vi "set_rep_param.vi"(4 "error in (no error)":errorcluster, 5 "par_val":string, 6 "param_name":string, 7 "refnum":T1) -> (0 "error out":errorcluster, 3 "refnum out":T1)   [LabVIEW 2010]
uses:
  <vilib>/Utility/config.llb/Config Data RefNum.ctl
  <vilib>/Utility/config.llb/Write Key (I32).vi
  <vilib>/Utility/config.llb/Write Key (String).vi
  <vilib>/Utility/config.llb/Read Key (String).vi
  <vilib>/Utility/config.llb/NI_LVConfig.lvlib
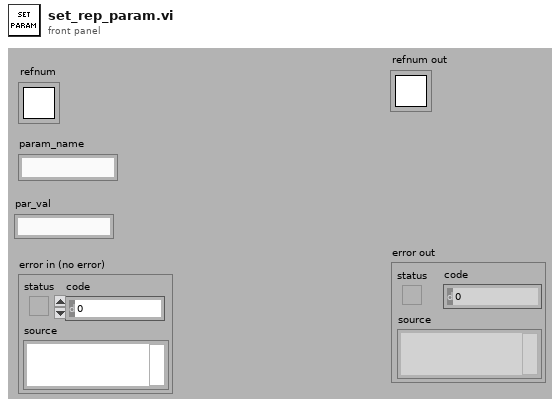
[diagram p1: front panel]
types:
  T1 = typedef "NI_LVConfig.lvlib/Config Data RefNum.ctl" = refnum<k1>
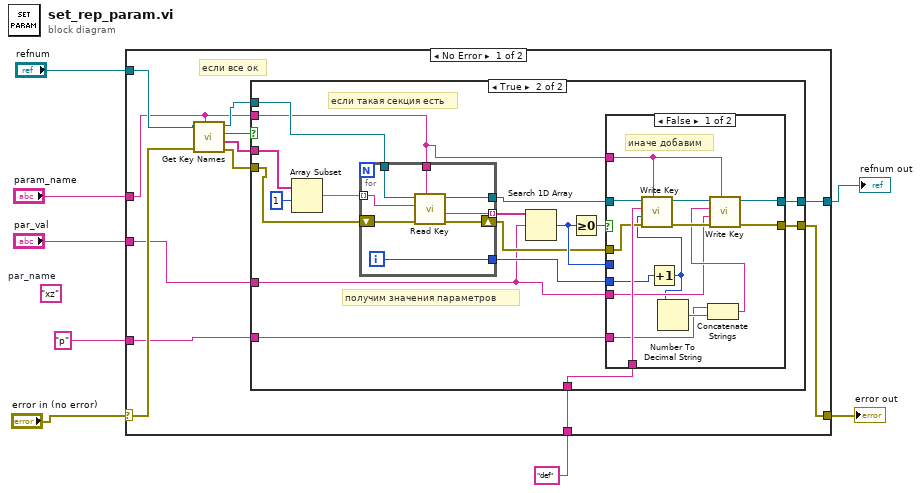
[diagram p0: block diagram]
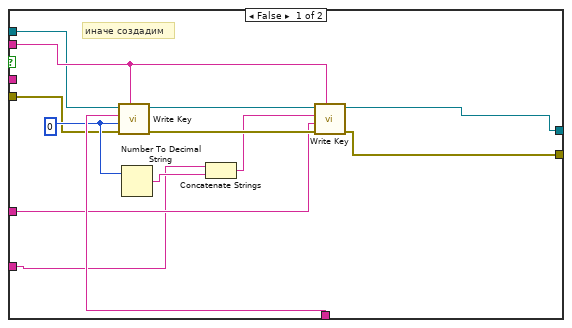
[diagram p2: hidden frame]
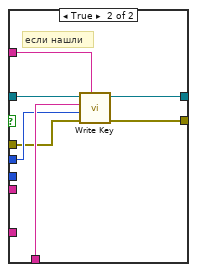
[diagram p3: hidden frame]
diagram:
  (unwired) "xz"  # par_name
  n1 = case shown="No Error" "error in (no error)" {
    selector: "error in (no error)" -> [w20 w81]
    tunnel: [w10 w81] -> w7
    tunnel: "refnum" -> [w19 w80]
    tunnel: "param_name" -> [w13 _]
    tunnel: "p" -> [w14 _]
    tunnel: "par_val" -> [w12 _]
    tunnel: "def" -> [w11 _]
    tunnel: [w9 w80] -> w1
    frame No Error {
      # "если все ок"
      n2 = call <vilib>:"Get Key Names.vi"("section"=w13, "error in (no error)"=w20, "refnum"=w19) -> ("error out"=w17:errorcluster, "key names"=w15:string[], "section exists?"=w18:bool, "refnum out"=w16:T1)  [unwired: 5 in]
      n3 = case shown="True" w18 {
        tunnel: w17 -> [w21 w48]
        tunnel: w16 -> [w30 w46]
        tunnel: w15 -> [_ w50]
        tunnel: w14 -> [w23 w37]
        tunnel: w13 -> [w31 w43]
        tunnel: w12 -> [w26 w36]
        tunnel: w11 -> [w27 w41]
        tunnel: [w28 w35] -> w10
        tunnel: [w29 w34] -> w9
        frame False {
          w25 = 0
          # "иначе создадим"
          n4 = call-poly <vilib>:"Write Key.vi"("section"=w31, "error in (no error)"=w21, "value"=w25, "key"=w27, "refnum"=w30) -> ("error out"=w33:errorcluster, "refnum out"=w32:T1)  [unwired: 4 in, 1 out]
          n5 = Number To Decimal String(number=w25) -> (decimal integer string=w24:string)  [unwired: 1 in]
          n6 = Concatenate Strings(w23, w24) -> (w22:string)
          n7 = call-poly <vilib>:"Write Key.vi"("section"=w31, "error in (no error)"=w33, "value"=w26, "key"=w22, "refnum"=w32) -> ("error out"=w28:errorcluster, "refnum out"=w29:T1)  [unwired: 4 in, 1 out]
        }
        frame True {
          # "получим значения параметров"
          # "если такая секция есть"
          n8 = Array Subset(array=w50, index=1) -> (w47:string[])  [unwired: 1 in]
          n9 = for {
            tunnel: w47 -> [w76] mode=indexing
            tunnel: w43 -> [w78]
            tunnel: w46 -> [w77]
            tunnel: [w74] -> w42
            tunnel: [w73] -> w45 mode=indexing
            shift-right: [w75] -> w39
            shift-left: w48 -> [w79]
            tunnel: [w72] -> w38
            i -> [w72]
            n10 = call-poly <vilib>:"Read Key.vi"("section"=w78, "error in (no error)"=w79, "key"=w76, "refnum"=w77) -> ("error out"=w75:errorcluster, "value"=w73:string, "refnum out"=w74:T1)  [unwired: 4 in, 1 out]
          }
          n11 = Search 1D Array(1D array=w45, element=w36) -> (index of element=w40:i32)  [unwired: 1 in]
          n12 = Greater Or Equal To 0?(x=w40) -> (x >= 0?=w44:bool)
          n13 = case shown="False" w44 {
            tunnel: w43 -> [w60 w71]
            tunnel: w42 -> [w62 w70]
            tunnel: w41 -> [w64 w69]
            tunnel: w40 -> [_ w68]
            tunnel: w39 -> [w63 w67]
            tunnel: [w59 w66] -> w35
            tunnel: [w58 w65] -> w34
            tunnel: w38 -> [w56 _]
            tunnel: w37 -> [w54 _]
            tunnel: w36 -> [w52 _]
            frame False {
              # "иначе добавим"
              n14 = Increment(x=w56) -> (x+1=w51:i32)
              n15 = call-poly <vilib>:"Write Key.vi"("section"=w60, "error in (no error)"=w63, "value"=w51, "key"=w64, "refnum"=w62) -> ("error out"=w61:errorcluster, "refnum out"=w57:T1)  [unwired: 4 in, 1 out]
              n16 = Number To Decimal String(number=w51) -> (decimal integer string=w55:string)  [unwired: 1 in]
              n17 = Concatenate Strings(w54, w55) -> (w53:string)
              n18 = call-poly <vilib>:"Write Key.vi"("section"=w60, "error in (no error)"=w61, "value"=w52, "key"=w53, "refnum"=w57) -> ("error out"=w59:errorcluster, "refnum out"=w58:T1)  [unwired: 4 in, 1 out]
            }
            frame True {
              # "если нашли"
              n19 = call-poly <vilib>:"Write Key.vi"("section"=w71, "error in (no error)"=w67, "value"=w68, "key"=w69, "refnum"=w70) -> ("error out"=w66:errorcluster, "refnum out"=w65:T1)  [unwired: 4 in, 1 out]
            }
          }
        }
      }
    }
    frame Error {
    }
  }
  "error out" <- w7
  "refnum out" <- w1
